vi "Get System Monitor Settings.vi"(8 "error in (no error)":errorcluster, 11 "Item Ref in":T2 format="%.0x") -> (0 "error out":errorcluster, 2 "System Monitor Settings":T1, 3 "Item Ref out":T2 format="%.0x")   [LabVIEW 2027, in "System Monitor System Explorer.lvlib"]
uses:
  System Monitor System Explorer.lvlib
  <vilib>/NI VeriStand/Custom Device API/Custom Device Item Ref.ctl
  Shared/System Monitor Settings.ctl
  Shared/Constants.vi
  <vilib>/NI VeriStand/Custom Device API/Get Item Property (U32).vi
  <vilib>/NI VeriStand/Custom Device API/Get Item Property (Double).vi
  <vilib>/NI VeriStand/Custom Device API/Custom Device API.lvlib
  Shared/System Monitor Shared.lvlib
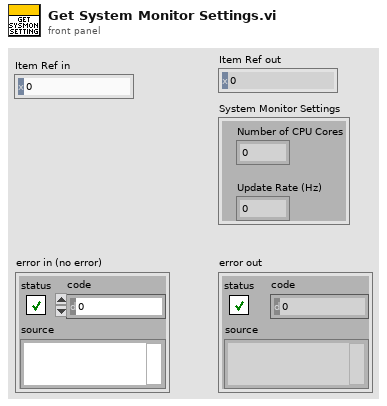
[diagram p1: front panel]
types:
  T1 = typedef "System Monitor Shared.lvlib/System Monitor Settings.ctl" = cluster{"Number of CPU Cores":u64, "Update Rate (Hz)":dbl}
  T2 = typedef "Custom Device API.lvlib/Custom Device Item Ref.ctl" = u64
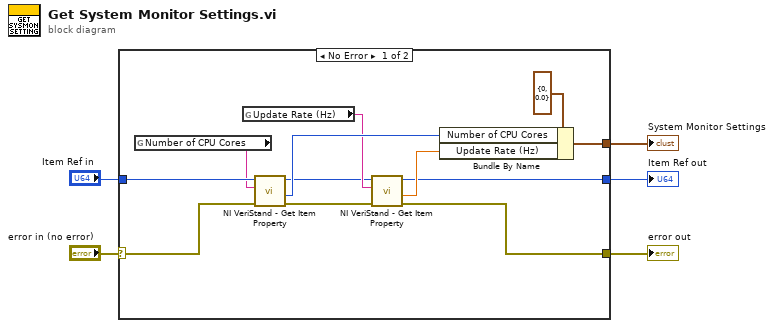
[diagram p0: block diagram]
diagram:
  n1 = case shown="No Error" "error in (no error)" {
    selector: "error in (no error)" -> [w16 w18]
    tunnel: [w7 w18] -> w2
    tunnel: "Item Ref in" -> [w17 w19]
    tunnel: [w6 w19] -> w4
    tunnel: [w13 _] -> w1
    frame No Error {
      n2 = global read "Constants.vi" "Number of CPU Cores"() -> (w15:string)
      n3 = global read "Constants.vi" "Update Rate (Hz)"() -> (w10:string)
      n4 = call-poly <vilib>:"NI VeriStand - Get Item Property.vi"("error in (no error)"=w16, "Property Name"=w15, "Item Ref in"=w17) -> ("error out"=w12:errorcluster, "Value"=w11:u32, "Item Ref out"=w9:T2)  [unwired: 5 in, 1 out]
      n5 = call-poly <vilib>:"NI VeriStand - Get Item Property.vi"("error in (no error)"=w12, "Property Name"=w10, "Item Ref in"=w9) -> ("error out"=w7:errorcluster, "Value"=w8:dbl, "Item Ref out"=w6:T2)  [unwired: 5 in, 1 out]
      n6 = Bundle By Name(cluster=T1 {"Number of CPU Cores"=0, "Update Rate (Hz)"=0.0} ("System Monitor Settings"), "Number of CPU Cores"=w11, "Update Rate (Hz)"=w8) -> (w13:T1)
    }
    frame Error {
    }
  }
  "Item Ref out" <- w4
  "System Monitor Settings" <- w1
  "error out" <- w2
